vi "prepare buffer array.vi"(7 "shots# per page":i32, 8 "error in (no error)":errorcluster, 9 "shot H":i32, 10 "page W":i32, 11 "buffer page #":i32) -> (0 "error out":errorcluster, 2 "Image array":T1[](array[typedef]), 3 "ptr array":u64[](array[numeric]))   [LabVIEW 2021, in "Camera.lvlib" / "Camera.lvclass"]
uses:
  Camera.lvclass
  <vilib>/vision/Image Controls.llb/IMAQ Image.ctl
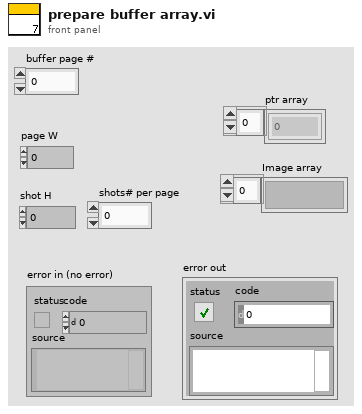
[diagram p1: front panel]
types:
  T1 = typedef "IMAQ Image.ctl" = refnum<image>
  T2 = enum32{"Map Pixel Pointer", "Unmap Pixel Pointer", "Get Pixels Infos"}
  T3 = typedef "Image Type" = u32
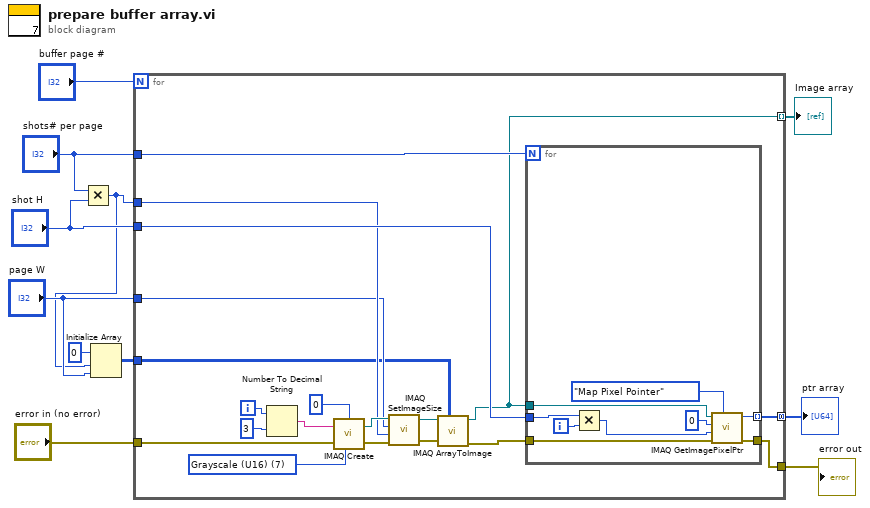
[diagram p0: block diagram]
diagram:
  n1 = Multiply(x="shots# per page", y="shot H") -> (x*y=w2:i32)
  n2 = Initialize Array(u16 0 ("element"), w2, "page W") -> (w1:u16[][])
  n3 = for {
    N: "buffer page #" -> [_]
    tunnel: "page W" -> [w13]
    tunnel: w2 -> [w14]
    tunnel: "error in (no error)" -> [w23]
    tunnel: "shots# per page" -> [w22]
    tunnel: "shot H" -> [w21]
    tunnel: [w20] -> w9 mode=concatenating
    tunnel: [w19] -> w8
    tunnel: [w17] -> w5 mode=indexing
    tunnel: w1 -> [w12]
    i -> [w29]
    w27 = T3 7 items=["Grayscale (U8)", "Grayscale (I16)", "Grayscale (SGL)", "Complex (CSG)", "RGB (U32)", "HSL (U32)", "RGB (U64)", "Grayscale (U16)"] ("Image Type")
    n4 = Number To Decimal String(number=w29, width (-)=i16 3) -> (decimal integer string=w26:string)
    n5 = call "IMAQ Create"("Border Size"=0, "Image Name"=w26, "Image Type"=w27, "error in (no error)"=w23) -> ("New Image"=w25:T1, "error out"=w24:errorcluster)  [unwired: 1 in]
    n6 = call "IMAQ SetImageSize"("error in (no error)"=w24, "Y Resolution"=w14, "X Resolution"=w13, "Image"=w25) -> ("error out"=w16:errorcluster, "Image Out"=w18:T1)  [unwired: 1 in]
    n7 = call "IMAQ ArrayToImage"("Image Pixels (U16)"=w12, "error in (no error)"=w16, "Image"=w18) -> ("error out"=w15:errorcluster, "Image Out"=w17:T1)  [unwired: 7 in]
    n8 = for {
      N: w22 -> [_]
      tunnel: w21 -> [w38]
      tunnel: w17 -> [w34]
      tunnel: w15 -> [w35]
      tunnel: [w32] -> w20 mode=indexing
      tunnel: [w31] -> w19
      i -> [w37]
      n9 = Multiply(x=w38, y=w37) -> (x*y=w36:i32)
      n10 = call "IMAQ GetImagePixelPtr"("Function"=T2."Map Pixel Pointer", "error in (no error)"=w35, "Y Coordinate"=w36, "X Coordinate"=0, "Image"=w34) -> ("error out"=w31:errorcluster, "Pixel Pointer out"=w32:u64)  [unwired: 1 in, 4 out]
    }
  }
  "ptr array" <- w9
  "error out" <- w8
  "Image array" <- w5
